vi "PCO_SetHWIOSignalTiming.vi"(0 "ph":u64, 5 "wSignalNum":u16, 7 "wSelect":u16, 9 "dwSignalTiming":u32, 11 "error in (no error)":errorcluster {"code" format="%x"}) -> (4 "ph out":u64, 6 "ErrorMessage":i32 format="%x", 15 "error out":errorcluster {"code" format="%x"})   [LabVIEW 2020, in "SDK.lvlib" / "TimingControl.lvlib"]
doc: "<b>Description:</b>\nSets the signal options of the requested signal number\nThis function call is optional. Please check camera description.\n\n<b>Supported camera type:</b>\npco.edge, pco.dimax\n\n<b>Descriptor dependency:</b>\ndwGeneralCapsDESC1: HW_IO_SIGNAL_DESCRIPTOR"
uses:
  TimingControl.lvlib
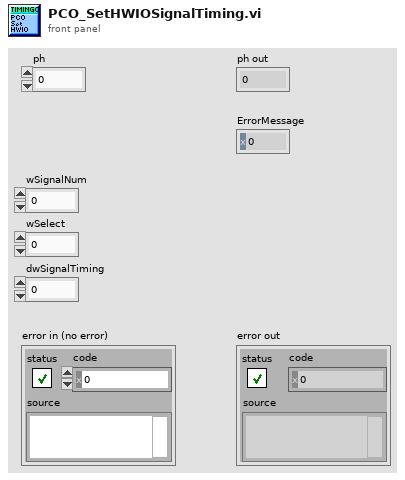
[diagram p1: front panel]
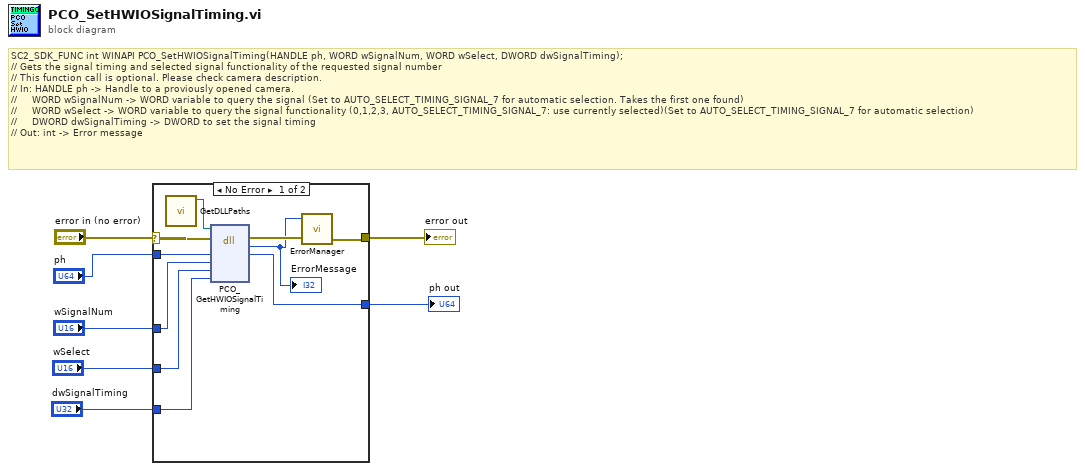
[diagram p0: block diagram]
diagram:
  # "SC2_SDK_FUNC int WINAPI PCO_SetHWIOSignalTiming(HANDLE ph, WORD wSignalNum, WORD wSelect, DWORD dwSignalTiming);\n// Gets the signal timing and selected signal functionality of the requested signal number\n// This function call is optional. Please check camera description.\n// In: HANDLE ph -> Handle to a proviously opened camera.\n//     WORD wSignalNum -> WORD variable to query the signal (Set to AUTO_SELECT_TIMING_SIGNAL_7 for automatic selection. Takes the first one found)\n//     WORD wSelect -> WORD variable to query the signal functionality (0,1,2,3, AUTO_SELECT_TIMING_SIGNAL_7: use currently selected)(Set to AUTO_SELECT_TIMING_SIGNAL_7 for automatic selection)\n//     DWORD dwSignalTiming -> DWORD to set the signal timing\n// Out: int -> Error message"
  n1 = case shown="No Error" "error in (no error)" {
    selector: "error in (no error)" -> [w12 w19]
    tunnel: "ph" -> [w17 w18]
    tunnel: [w16 w18] -> w6
    tunnel: [w14 w19] -> w5
    tunnel: "wSignalNum" -> [w10 _]
    tunnel: "wSelect" -> [w9 _]
    tunnel: "dwSignalTiming" -> [w8 _]
    frame No Error {
      n2 = call "GetDLLPaths.vi"() -> ("SC2_Cam_Path"=w11:path)  [unwired: 9 in, 2 out]
      n3 = dll-call lib="?" fn="PCO_GetHWIOSignalTiming"(path in=w11, error in=w12, "ph"=w17, "wSignalNum"=w10, "wSelect"=w9, "dwSignalTiming"=w8) -> (error out=w15:errorcluster, "return type"=w13:i32, "ph"=w16:u64)  [unwired: 4 in, 1 out]
      "ErrorMessage" <- w13
      n4 = call "ErrorManager.vi"("error in (no error)"=w15, "error code"=w13) -> ("error out"=w14:errorcluster)  [unwired: 3 in]
    }
    frame Error {
    }
  }
  "ph out" <- w6
  "error out" <- w5
